vi "QMH_ICR_Control_EnQueue.vi"(7 "Last ?":bool, 8 "error in (no error)":errorcluster caption="entrée d'erreur (pas d'erreur)", 9 "Variant":variant, 10 "Command":T1, 11 "ICR Queue":refnum<queue>) -> (0 "error out":errorcluster caption="sortie d'erreur", 3 "ICR Queue":refnum<queue>)   [LabVIEW 2020]
uses:
  controls/QMH_ICR_Message.ctl
  controls/QMH_ICR_Command.ctl
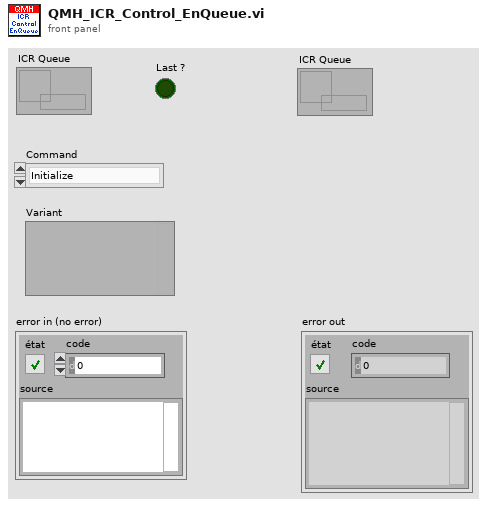
[diagram p1: front panel]
types:
  T1 = typedef "QMH_ICR_Command.ctl" = enum16{"Initialize", "Sequence Loop Setup", "Sequence Setup", "ICR Start", "ICR Stop", "Hardware Setup", "Next Sequence Loop", "Next Accumulation", "Waiting for Trigger", "Sequence Started", "Sequence Finished", "Sequence Loop Done", "Writing Data", "Hardware Reset", "Exit"}
  T2 = typedef "QMH_ICR_Message.ctl" = cluster{"Command":T1, "Data":variant}
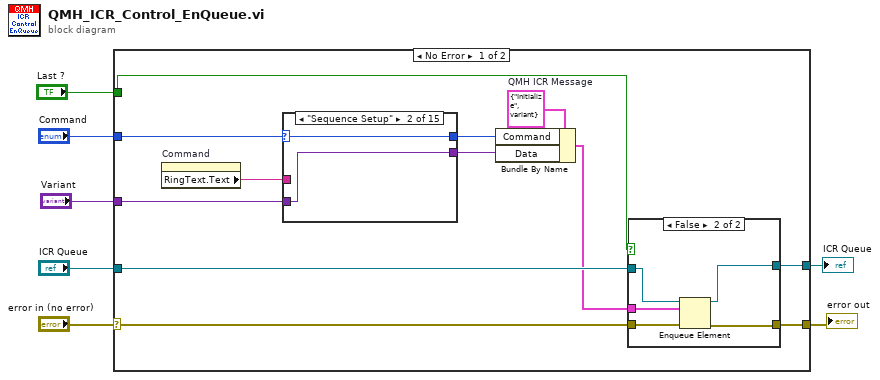
[diagram p0: block diagram]
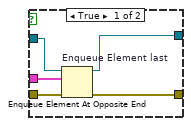
[diagram p2: hidden frame]
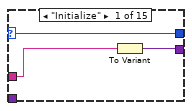
[diagram p3: hidden frame]
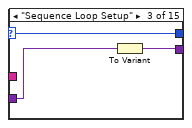
[diagram p4: hidden frame]
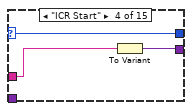
[diagram p5: hidden frame]
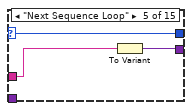
[diagram p6: hidden frame]
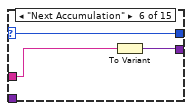
[diagram p7: hidden frame]
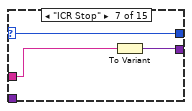
[diagram p8: hidden frame]
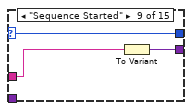
[diagram p10: hidden frame]
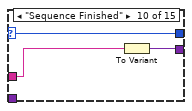
[diagram p11: hidden frame]
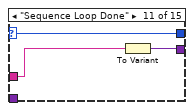
[diagram p12: hidden frame]
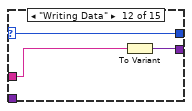
[diagram p13: hidden frame]
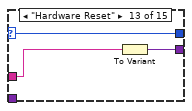
[diagram p14: hidden frame]
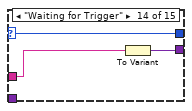
[diagram p15: hidden frame]
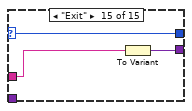
[diagram p16: hidden frame]
diagram:
  n1 = case shown="No Error" "error in (no error)" {
    selector: "error in (no error)" -> [w17 w73]
    tunnel: [w16 w73] -> w6
    tunnel: "ICR Queue" -> [w19 _]
    tunnel: [w18 _] -> w1
    tunnel: "Command" -> [w15 _]
    tunnel: "Variant" -> [w13 _]
    tunnel: "Last ?" -> [w10 _]
    frame No Error {
      w9 = T2 {"Command"=enum."Initialize", "Data"=variant}  # QMH ICR Message
      n2 = property on="Command" class="Enum (strict)"() -> ("RingText.Text"=w11:string)  [unwired: 2 in, 2 out]
      n3 = case shown="\"Sequence Setup\"" w15 {
        selector: w15 -> [w32 w34 w37 w40 w43 w46 w49 w51 w54 w57 w60 w63 w66 w69 w72]
        tunnel: [w31 w33 w36 w39 w42 w45 w48 w50 w52 w55 w58 w62 w64 w68 w71] -> w12
        tunnel: [w32 w34 w37 w40 w43 w46 w49 w51 w54 w57 w60 w63 w66 w69 w72] -> w14
        tunnel: w13 -> [_ w33 w35 _ _ _ _ w50 _ _ _ _ _ _ _]
        tunnel: w11 -> [w30 _ _ w38 w41 w44 w47 _ w53 w56 w59 w61 w65 w67 w70]
        frame "Initialize" {
          n4 = To Variant(anything=w30) -> (Variant=w31:variant)
        }
        frame "Sequence Setup" {
        }
        frame "Sequence Loop Setup" {
          n5 = To Variant(anything=w35) -> (Variant=w36:variant)
        }
        frame "ICR Start" {
          n6 = To Variant(anything=w38) -> (Variant=w39:variant)
        }
        frame "Next Sequence Loop" {
          n7 = To Variant(anything=w41) -> (Variant=w42:variant)
        }
        frame "Next Accumulation" {
          n8 = To Variant(anything=w44) -> (Variant=w45:variant)
        }
        frame "ICR Stop" {
          n9 = To Variant(anything=w47) -> (Variant=w48:variant)
        }
        frame "Hardware Setup" {
        }
        frame "Sequence Started" {
          n10 = To Variant(anything=w53) -> (Variant=w52:variant)
        }
        frame "Sequence Finished" {
          n11 = To Variant(anything=w56) -> (Variant=w55:variant)
        }
        frame "Sequence Loop Done" {
          n12 = To Variant(anything=w59) -> (Variant=w58:variant)
        }
        frame "Writing Data" {
          n13 = To Variant(anything=w61) -> (Variant=w62:variant)
        }
        frame "Hardware Reset" {
          n14 = To Variant(anything=w65) -> (Variant=w64:variant)
        }
        frame "Waiting for Trigger" {
          n15 = To Variant(anything=w67) -> (Variant=w68:variant)
        }
        frame "Exit" {
          n16 = To Variant(anything=w70) -> (Variant=w71:variant)
        }
      }
      n17 = Bundle By Name(cluster=w9, "Command"=w14, "Data"=w12) -> (w8:T2)
      n18 = case shown="False" w10 {
        tunnel: w19 -> [w21 w27]
        tunnel: [w20 w26] -> w18
        tunnel: w17 -> [w24 w29]
        tunnel: [w23 w28] -> w16
        tunnel: w8 -> [w22 w25]
        frame True {
          n19 = Enqueue Element At Opposite End "Enqueue Element last"(queue=w21, element=w22, error in (no error)=w24) -> (queue out=w20:refnum<queue>, error out=w23:errorcluster)  [unwired: 1 in, 1 out]
        }
        frame False {
          n20 = Enqueue Element(queue=w27, element=w25, error in (no error)=w29) -> (queue out=w26:refnum<queue>, error out=w28:errorcluster)  [unwired: 1 in, 1 out]
        }
      }
    }
    frame Error {
    }
  }
  "error out" <- w6
  "ICR Queue" <- w1
